vi "WILT Water Valve Control.vi"(0 "Valve Status":T7, 2 "Station Group":T4, 3 "Station Number":u32, 5 "Error In":errorcluster, 8 "Agilent Valve and Switch Locations":T3[](array[typedef])=[{"Channel"="301", "Station"="1", "Label"="Water Valve", "Agilent Station"="2", "Data"=0.0}, {"Channel"="302", "Station"="2", "Label"="Water Valve", "Agilent Station"="2", "Data"=0.0}, {"Channel"="303", "Station"="3", "Label"="Water Valve", "Agilent Station"="2", "Data"=0.0}, {"Channel"="304", "Station"="4", "Label"="Water Valve", "Agilent Station"="2", "Data"=0.0}, {"Channel"="305", "Station"="5", "Label"="Water Valve", "Agilent Station"="2", "Data"=0.0}, {"Channel"="306", "Station"="6", "Label"="Water Valve", "Agilent Station"="2", "Data"=0.0}, {"Channel"="307", "Station"="7", "Label"="Water Valve", "Agilent Station"="2", "Data"=0.0}, {"Channel"="308", "Station"="8", "Label"="Water Valve", "Agilent Station"="2", "Data"=0.0}, {"Channel"="309", "Station"="9", "Label"="Water Valve", "Agilent Station"="2", "Data"=0.0}, {"Channel"="310", "Station"="10", "Label"="Water Valve", "Agilent Station"="2", "Data"=0.0}, {"Channel"="311", "Station"="11", "Label"="Water Valve", "Agilent Station"="2", "Data"=0.0}, {"Channel"="312", "Station"="12", "Label"="Water Valve", "Agilent Station"="2", "Data"=0.0}, {"Channel"="313", "Station"="13", "Label"="Water Valve", "Agilent Station"="2", "Data"=0.0}, {"Channel"="314", "Station"="14", "Label"="Water Valve", "Agilent Station"="2", "Data"=0.0}, {"Channel"="315", "Station"="15", "Label"="Water Valve", "Agilent Station"="2", "Data"=0.0}, {"Channel"="316", "Station"="16", "Label"="Water Valve", "Agilent Station"="2", "Data"=0.0}, {"Channel"="317", "Station"="17", "Label"="Water Valve", "Agilent Station"="2", "Data"=0.0}, {"Channel"="318", "Station"="18", "Label"="Water Valve", "Agilent Station"="2", "Data"=0.0}, {"Channel"="319", "Station"="19", "Label"="Water Valve", "Agilent Station"="2", "Data"=0.0}, {"Channel"="320", "Station"="20", "Label"="Water Valve", "Agilent Station"="2", "Data"=0.0}, {"Channel"="101", "Station"="21", "Label"="Water Valve", "Agilent Station"="3", "Data"=0.0}, {"Channel"="102", "Station"="22", "Label"="Water Valve", "Agilent Station"="3", "Data"=0.0}, {"Channel"="103", "Station"="23", "Label"="Water Valve", "Agilent Station"="3", "Data"=0.0}, {"Channel"="104", "Station"="24", "Label"="Water Valve", "Agilent Station"="3", "Data"=0.0}, {"Channel"="105", "Station"="25", "Label"="Water Valve", "Agilent Station"="3", "Data"=0.0}, {"Channel"="106", "Station"="26", "Label"="Water Valve", "Agilent Station"="3", "Data"=0.0}, {"Channel"="107", "Station"="27", "Label"="Water Valve", "Agilent Station"="3", "Data"=0.0}, {"Channel"="108", "Station"="28", "Label"="Water Valve", "Agilent Station"="3", "Data"=0.0}, {"Channel"="109", "Station"="29", "Label"="Water Valve", "Agilent Station"="3", "Data"=0.0}, {"Channel"="110", "Station"="30", "Label"="Water Valve", "Agilent Station"="3", "Data"=0.0}, {"Channel"="111", "Station"="31", "Label"="Water Valve", "Agilent Station"="3", "Data"=0.0}, {"Channel"="112", "Station"="32", "Label"="Water Valve", "Agilent Station"="3", "Data"=0.0}, {"Channel"="101", "Station"="33", "Label"="Water Valve", "Agilent Station"="5", "Data"=0.0}, {"Channel"="102", "Station"="34", "Label"="Water Valve", "Agilent Station"="5", "Data"=0.0}, {"Channel"="103", "Station"="35", "Label"="Water Valve", "Agilent Station"="5", "Data"=0.0}, {"Channel"="104", "Station"="36", "Label"="Water Valve", "Agilent Station"="5", "Data"=0.0}, {"Channel"="105", "Station"="37", "Label"="Water Valve", "Agilent Station"="5", "Data"=0.0}, {"Channel"="106", "Station"="38", "Label"="Water Valve", "Agilent Station"="5", "Data"=0.0}, {"Channel"="107", "Station"="39", "Label"="Water Valve", "Agilent Station"="5", "Data"=0.0}, {"Channel"="108", "Station"="40", "Label"="Water Valve", "Agilent Station"="5", "Data"=0.0}, {"Channel"="109", "Station"="41", "Label"="Water Valve", "Agilent Station"="5", "Data"=0.0}, {"Channel"="110", "Station"="42", "Label"="Water Valve", "Agilent Station"="5", "Data"=0.0}, {"Channel"="111", "Station"="43", "Label"="Water Valve", "Agilent Station"="5", "Data"=0.0}, {"Channel"="112", "Station"="44", "Label"="Water Valve", "Agilent Station"="5", "Data"=0.0}, {"Channel"="113", "Station"="45", "Label"="Water Valve", "Agilent Station"="5", "Data"=0.0}, {"Channel"="114", "Station"="46", "Label"="Water Valve", "Agilent Station"="5", "Data"=0.0}, {"Channel"="115", "Station"="47", "Label"="Water Valve", "Agilent Station"="5", "Data"=0.0}, {"Channel"="116", "Station"="48", "Label"="Water Valve", "Agilent Station"="5", "Data"=0.0}, {"Channel"="117", "Station"="49", "Label"="Water Valve", "Agilent Station"="5", "Data"=0.0}, {"Channel"="118", "Station"="50", "Label"="Water Valve", "Agilent Station"="5", "Data"=0.0}, {"Channel"="119", "Station"="51", "Label"="Water Valve", "Agilent Station"="5", "Data"=0.0}, {"Channel"="120", "Station"="52", "Label"="Water Valve", "Agilent Station"="5", "Data"=0.0}, {"Channel"="201", "Station"="53", "Label"="Water Valve", "Agilent Station"="5", "Data"=0.0}, {"Channel"="202", "Station"="54", "Label"="Water Valve", "Agilent Station"="5", "Data"=0.0}, {"Channel"="203", "Station"="55", "Label"="Water Valve", "Agilent Station"="5", "Data"=0.0}, {"Channel"="204", "Station"="56", "Label"="Water Valve", "Agilent Station"="5", "Data"=0.0}, {"Channel"="301", "Station"="21", "Label"="Start Button", "Agilent Station"="5", "Data"=0.0}, {"Channel"="302", "Station"="22", "Label"="Start Button", "Agilent Station"="5", "Data"=0.0}, {"Channel"="303", "Station"="23", "Label"="Start Button", "Agilent Station"="5", "Data"=0.0}, {"Channel"="304", "Station"="24", "Label"="Start Button", "Agilent Station"="5", "Data"=0.0}, {"Channel"="305", "Station"="25", "Label"="Start Button", "Agilent Station"="5", "Data"=0.0}, {"Channel"="306", "Station"="26", "Label"="Start Button", "Agilent Station"="5", "Data"=0.0}, {"Channel"="307", "Station"="27", "Label"="Start Button", "Agilent Station"="5", "Data"=0.0}, {"Channel"="308", "Station"="28", "Label"="Start Button", "Agilent Station"="5", "Data"=0.0}, {"Channel"="309", "Station"="29", "Label"="Start Button", "Agilent Station"="5", "Data"=0.0}, {"Channel"="310", "Station"="30", "Label"="Start Button", "Agilent Station"="5", "Data"=0.0}, {"Channel"="311", "Station"="31", "Label"="Start Button", "Agilent Station"="5", "Data"=0.0}, {"Channel"="312", "Station"="32", "Label"="Start Button", "Agilent Station"="5", "Data"=0.0}, {"Channel"="101", "Station"="33", "Label"="Start Button", "Agilent Station"="7", "Data"=0.0}, {"Channel"="102", "Station"="34", "Label"="Start Button", "Agilent Station"="7", "Data"=0.0}, {"Channel"="103", "Station"="35", "Label"="Start Button", "Agilent Station"="7", "Data"=0.0}, {"Channel"="104", "Station"="36", "Label"="Start Button", "Agilent Station"="7", "Data"=0.0}, {"Channel"="105", "Station"="37", "Label"="Start Button", "Agilent Station"="7", "Data"=0.0}, {"Channel"="106", "Station"="38", "Label"="Start Button", "Agilent Station"="7", "Data"=0.0}, {"Channel"="107", "Station"="39", "Label"="Start Button", "Agilent Station"="7", "Data"=0.0}, {"Channel"="108", "Station"="40", "Label"="Start Button", "Agilent Station"="7", "Data"=0.0}, {"Channel"="109", "Station"="41", "Label"="Start Button", "Agilent Station"="7", "Data"=0.0}, {"Channel"="110", "Station"="42", "Label"="Start Button", "Agilent Station"="7", "Data"=0.0}, {"Channel"="111", "Station"="43", "Label"="Start Button", "Agilent Station"="7", "Data"=0.0}, {"Channel"="112", "Station"="44", "Label"="Start Button", "Agilent Station"="7", "Data"=0.0}, {"Channel"="113", "Station"="45", "Label"="Start Button", "Agilent Station"="7", "Data"=0.0}, {"Channel"="114", "Station"="46", "Label"="Start Button", "Agilent Station"="7", "Data"=0.0}, {"Channel"="115", "Station"="47", "Label"="Start Button", "Agilent Station"="7", "Data"=0.0}, {"Channel"="116", "Station"="48", "Label"="Start Button", "Agilent Station"="7", "Data"=0.0}, {"Channel"="117", "Station"="49", "Label"="Start Button", "Agilent Station"="7", "Data"=0.0}, {"Channel"="118", "Station"="50", "Label"="Start Button", "Agilent Station"="7", "Data"=0.0}, {"Channel"="119", "Station"="51", "Label"="Start Button", "Agilent Station"="7", "Data"=0.0}, {"Channel"="120", "Station"="52", "Label"="Start Button", "Agilent Station"="7", "Data"=0.0}, {"Channel"="201", "Station"="53", "Label"="Start Button", "Agilent Station"="7", "Data"=0.0}, {"Channel"="202", "Station"="54", "Label"="Start Button", "Agilent Station"="7", "Data"=0.0}, {"Channel"="203", "Station"="55", "Label"="Start Button", "Agilent Station"="7", "Data"=0.0}, {"Channel"="204", "Station"="56", "Label"="Start Button", "Agilent Station"="7", "Data"=0.0}], 9 "Step 3 Input in":T5, 11 "Day/Night Cycle":T2, 13 "Semaphore":T1[](array[typedef])) -> (14 "Step 3 Input out":T5, 19 "Error Out":errorcluster)   [LabVIEW 2016]
uses:
  Type Definitions/WILT Water Valve Control.ctl
  Type Definitions/WILT Station Test State Cluster.ctl
  Type Definitions/WILT Dryer Test State.ctl
  Type Definitions/WILT Room Location.ctl
  Type Definitions/WILT Agilent Channel Definition.ctl
  Type Definitions/WILT Day Night Cycle Enum.ctl
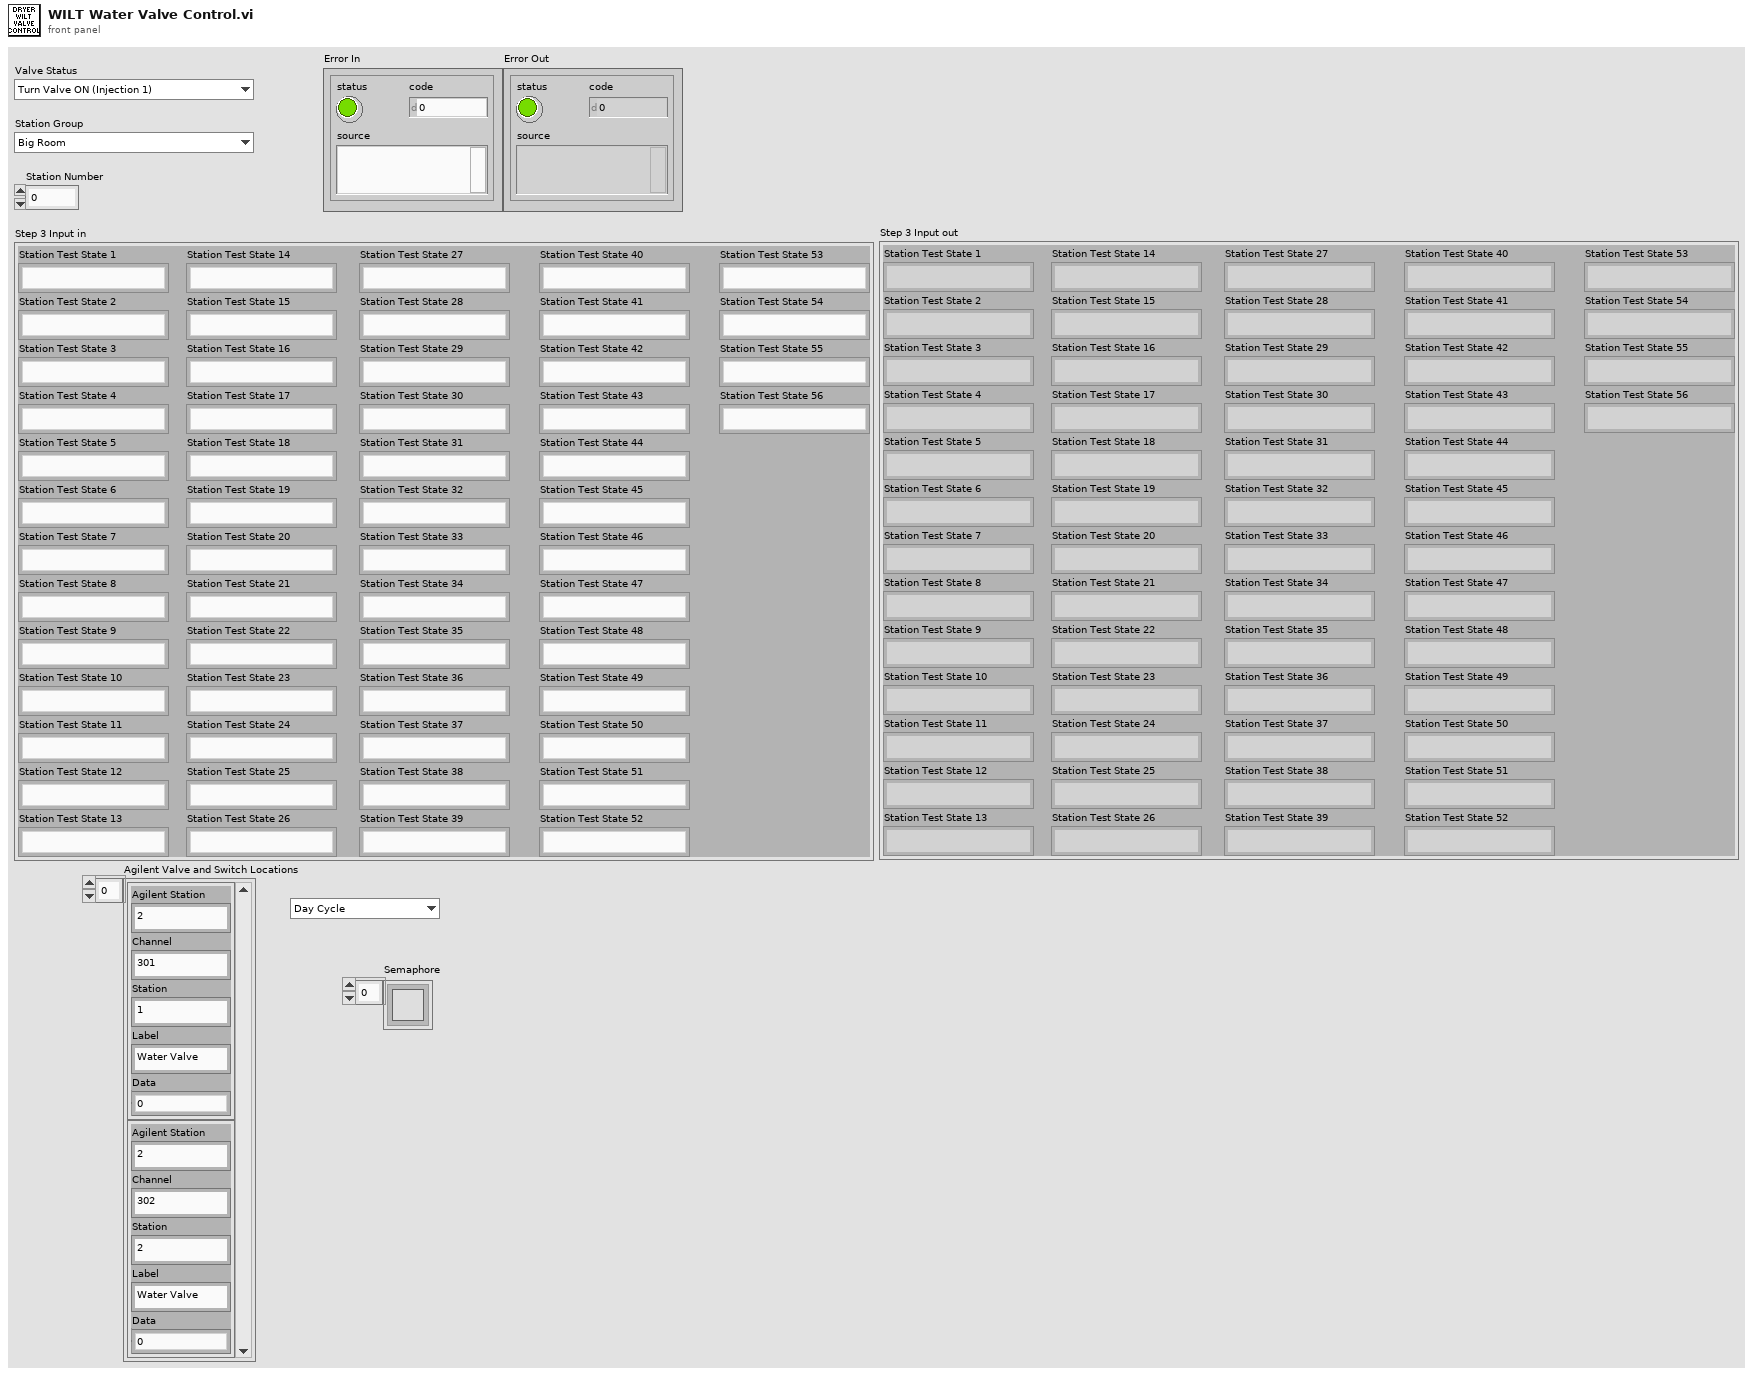
[diagram p1: front panel]
types:
  T1 = typedef "Semaphore RefNum" = refnum<k1>
  T2 = typedef "WILT Day Night Cycle Enum.ctl" = enum16{"Day Cycle", "Night Cycle", "Day Cycle (No Water)"}
  T3 = typedef "WILT Agilent Channel Definition.ctl" = cluster{"Channel":string, "Station":string, "Label":string, "Agilent Station":string, "Data":dbl}
  T4 = typedef "WILT Room Location.ctl" = enum16{"Big Room", "Remote Stations"}
  T5 = typedef "WILT Station Test State Cluster.ctl" = cluster{"Station Test State 1":T6, "Station Test State 2":T6, "Station Test State 3":T6, "Station Test State 4":T6, "Station Test State 5":T6, "Station Test State 6":T6, "Station Test State 7":T6, "Station Test State 8":T6, "Station Test State 9":T6, "Station Test State 10":T6, "Station Test State 11":T6, "Station Test State 12":T6, "Station Test State 13":T6, "Station Test State 14":T6, "Station Test State 15":T6, "Station Test State 16":T6, "Station Test State 17":T6, "Station Test State 18":T6, "Station Test State 19":T6, "Station Test State 20":T6, "Station Test State 21":T6, "Station Test State 22":T6, "Station Test State 23":T6, "Station Test State 24":T6, "Station Test State 25":T6, "Station Test State 26":T6, "Station Test State 27":T6, "Station Test State 28":T6, "Station Test State 29":T6, "Station Test State 30":T6, "Station Test State 31":T6, "Station Test State 32":T6, "Station Test State 33":T6, "Station Test State 34":T6, "Station Test State 35":T6, "Station Test State 36":T6, "Station Test State 37":T6, "Station Test State 38":T6, "Station Test State 39":T6, "Station Test State 40":T6, "Station Test State 41":T6, "Station Test State 42":T6, "Station Test State 43":T6, "Station Test State 44":T6, "Station Test State 45":T6, "Station Test State 46":T6, "Station Test State 47":T6, "Station Test State 48":T6, "Station Test State 49":T6, "Station Test State 50":T6, "Station Test State 51":T6, "Station Test State 52":T6, "Station Test State 53":T6, "Station Test State 54":T6, "Station Test State 55":T6, "Station Test State 56":T6}
  T6 = typedef "WILT Dryer Test State.ctl" = enum16{"No Serial Number", "Waiting for Dryer To Start", "Drying Clothes", "Water Injection 1 (On)", "Water Injection 1 Timer", "Water Injection 1 (Off)", "Pause Dryer", "Sending Start Stop CMD", "Pause Dryer 2", "Sending Start Stop CMD 2", "Drying Clothes 2", "Water Injection 2 (On)", "Water Injection 2 Timer", "Water Injection 2 (Off)", "Drying Clothes 3", "Cooling Down", "Sending Start Stop CMD 3", "Increment Cycle"}
  T7 = typedef "WILT Water Valve Control.ctl" = enum16{"Turn Valve ON (Injection 1)", "Turn Valve OFF (Injection 1)", "Turn Valve ON (Injection 2)", "Turn Valve OFF (Injection 2)"}
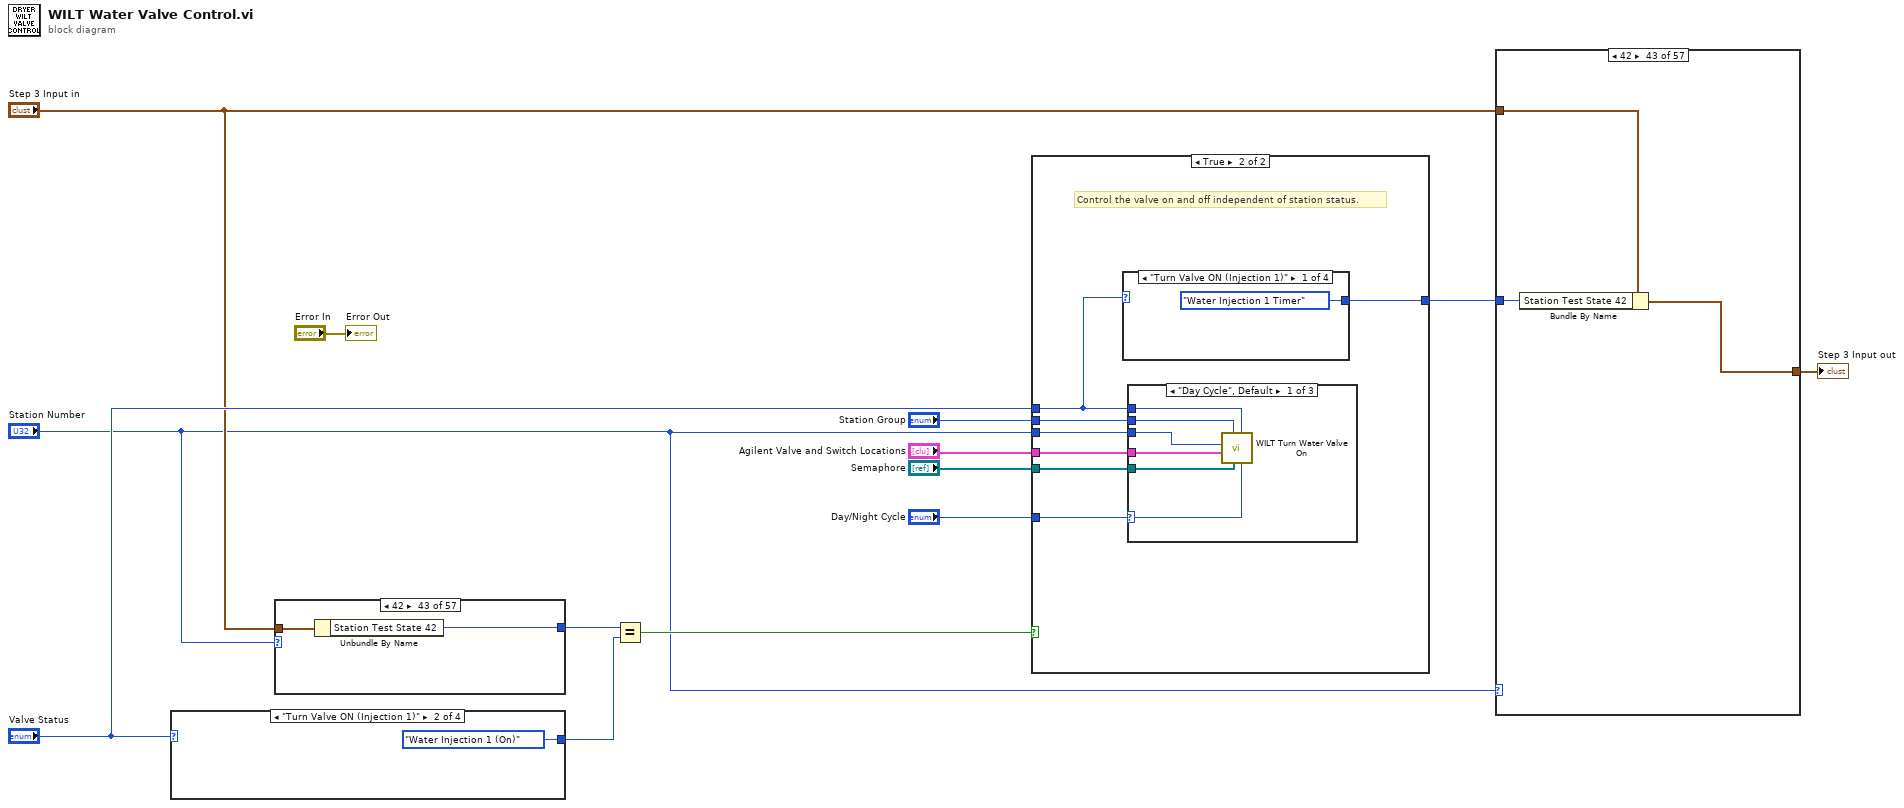
[diagram p0: block diagram]
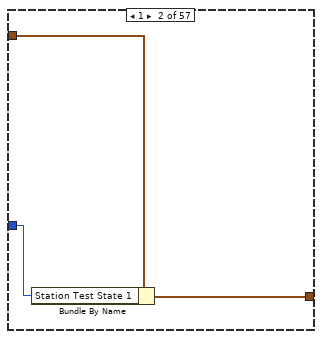
[diagram p3: hidden frame]
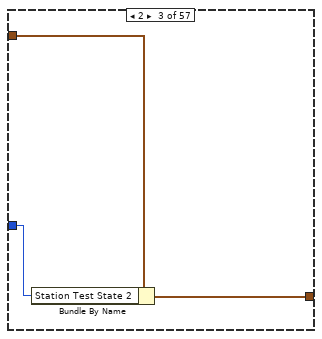
[diagram p4: hidden frame]
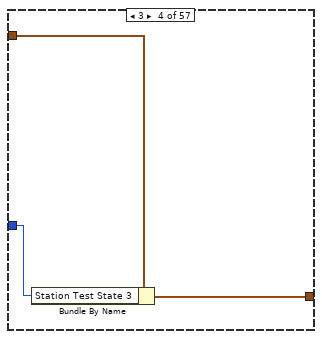
[diagram p5: hidden frame]
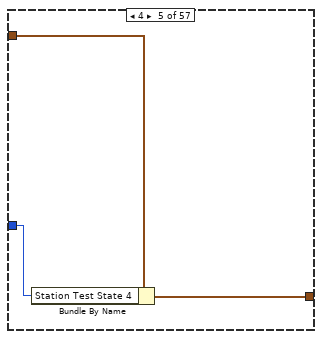
[diagram p6: hidden frame]
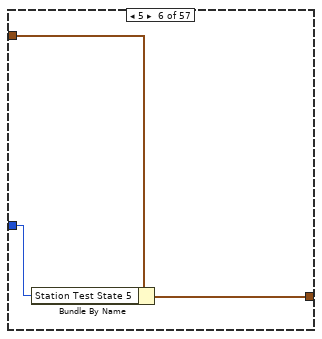
[diagram p7: hidden frame]
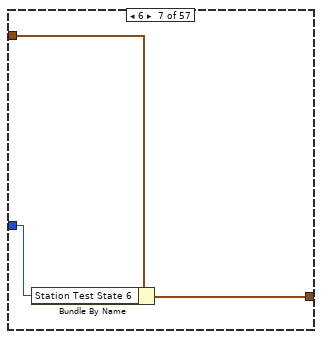
[diagram p8: hidden frame]
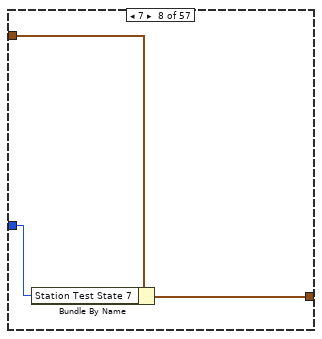
[diagram p9: hidden frame]
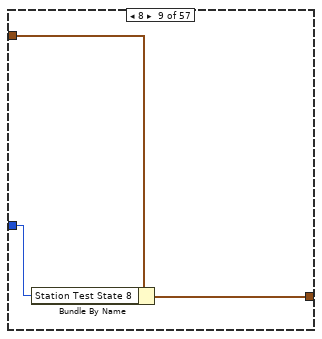
[diagram p10: hidden frame]
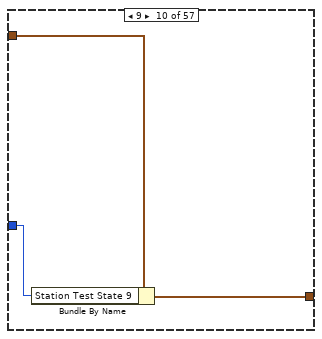
[diagram p11: hidden frame]
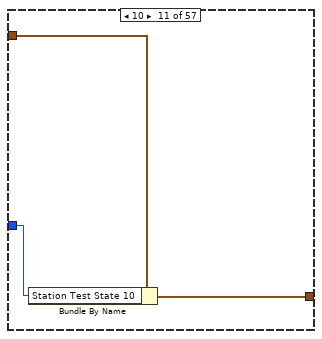
[diagram p12: hidden frame]
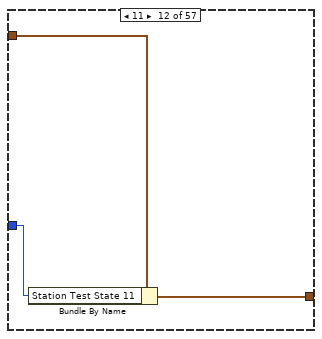
[diagram p13: hidden frame]
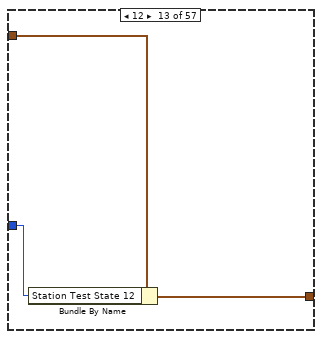
[diagram p14: hidden frame]
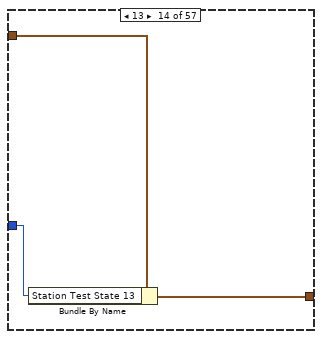
[diagram p15: hidden frame]
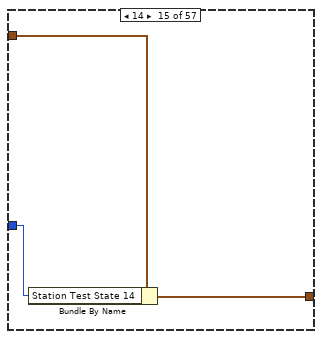
[diagram p16: hidden frame]
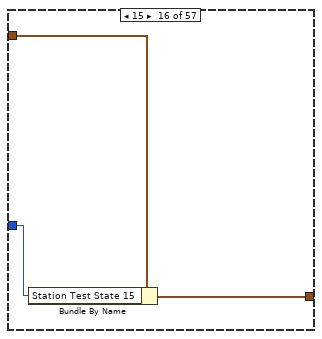
[diagram p17: hidden frame]
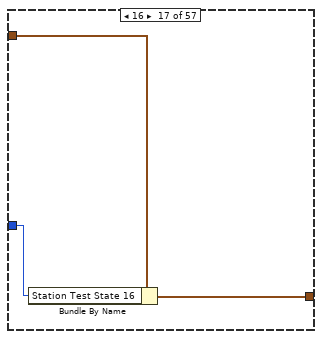
[diagram p18: hidden frame]
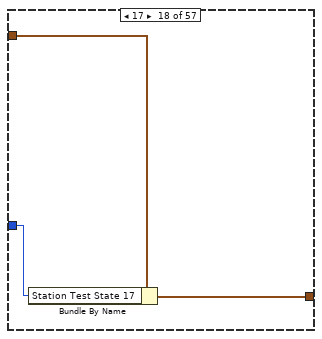
[diagram p19: hidden frame]
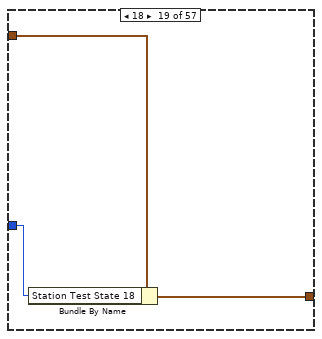
[diagram p20: hidden frame]
diagram:
  n1 = case shown="\"Turn Valve ON (Injection 1)\"" "Valve Status" {
    tunnel: [WILT_Dryer_Test_State."Water Injection 1 (Off)" ("y") WILT_Dryer_Test_State."Water Injection 1 (On)" ("y") WILT_Dryer_Test_State."Water Injection 2 (On)" ("y") WILT_Dryer_Test_State."Water Injection 2 (Off)" ("y")] -> w10
    frame "Turn Valve OFF (Injection 1)", Default {
    }
    frame "Turn Valve ON (Injection 1)" {
    }
    frame "Turn Valve ON (Injection 2)" {
    }
    frame "Turn Valve OFF (Injection 2)" {
    }
  }
  n2 = case shown="42" "Station Number" {
    tunnel: "Step 3 Input in" -> [_ w20 w22 w24 w26 w28 w30 w32 w34 w36 w38 w40 w42 w44 w46 w48 w50 w52 w54 w56 w58 w60 w62 w64 w66 w68 w70 w72 w74 w76 w78 w80 w82 w84 w86 w88 w90 w92 w94 w96 w98 w100 w102 w104 w106 w108 w110 w112 w114 w116 w118 w120 w122 w124 w126 w128 w130]
    tunnel: [WILT_Dryer_Test_State."No Serial Number" ("Station Test State 56") w19 w21 w23 w25 w27 w29 w31 w33 w35 w37 w39 w41 w43 w45 w47 w49 w51 w53 w55 w57 w59 w61 w63 w65 w67 w69 w71 w73 w75 w77 w79 w81 w83 w85 w87 w89 w91 w93 w95 w97 w99 w101 w103 w105 w107 w109 w111 w113 w115 w117 w119 w121 w123 w125 w127 w129] -> w9
    frame 0, Default {
      # "This is not a station.\nDo nothing"
    }
    frame 1 {
      n3 = Unbundle By Name(w20) -> ("Station Test State 1"=w19:T6)
    }
    frame 2 {
      n4 = Unbundle By Name(w22) -> ("Station Test State 2"=w21:T6)
    }
    frame 3 {
      n5 = Unbundle By Name(w24) -> ("Station Test State 3"=w23:T6)
    }
    frame 4 {
      n6 = Unbundle By Name(w26) -> ("Station Test State 4"=w25:T6)
    }
    frame 5 {
      n7 = Unbundle By Name(w28) -> ("Station Test State 5"=w27:T6)
    }
    frame 6 {
      n8 = Unbundle By Name(w30) -> ("Station Test State 6"=w29:T6)
    }
    frame 7 {
      n9 = Unbundle By Name(w32) -> ("Station Test State 7"=w31:T6)
    }
    frame 8 {
      n10 = Unbundle By Name(w34) -> ("Station Test State 8"=w33:T6)
    }
    frame 9 {
      n11 = Unbundle By Name(w36) -> ("Station Test State 9"=w35:T6)
    }
    frame 10 {
      n12 = Unbundle By Name(w38) -> ("Station Test State 10"=w37:T6)
    }
    frame 11 {
      n13 = Unbundle By Name(w40) -> ("Station Test State 11"=w39:T6)
    }
    frame 12 {
      n14 = Unbundle By Name(w42) -> ("Station Test State 12"=w41:T6)
    }
    frame 13 {
      n15 = Unbundle By Name(w44) -> ("Station Test State 13"=w43:T6)
    }
    frame 14 {
      n16 = Unbundle By Name(w46) -> ("Station Test State 14"=w45:T6)
    }
    frame 15 {
      n17 = Unbundle By Name(w48) -> ("Station Test State 15"=w47:T6)
    }
    frame 16 {
      n18 = Unbundle By Name(w50) -> ("Station Test State 16"=w49:T6)
    }
    frame 17 {
      n19 = Unbundle By Name(w52) -> ("Station Test State 17"=w51:T6)
    }
    frame 18 {
      n20 = Unbundle By Name(w54) -> ("Station Test State 18"=w53:T6)
    }
    frame 19 {
      n21 = Unbundle By Name(w56) -> ("Station Test State 19"=w55:T6)
    }
    frame 20 {
      n22 = Unbundle By Name(w58) -> ("Station Test State 20"=w57:T6)
    }
    frame 21 {
      n23 = Unbundle By Name(w60) -> ("Station Test State 21"=w59:T6)
    }
    frame 22 {
      n24 = Unbundle By Name(w62) -> ("Station Test State 22"=w61:T6)
    }
    frame 23 {
      n25 = Unbundle By Name(w64) -> ("Station Test State 23"=w63:T6)
    }
    frame 24 {
      n26 = Unbundle By Name(w66) -> ("Station Test State 24"=w65:T6)
    }
    frame 25 {
      n27 = Unbundle By Name(w68) -> ("Station Test State 25"=w67:T6)
    }
    frame 26 {
      n28 = Unbundle By Name(w70) -> ("Station Test State 26"=w69:T6)
    }
    frame 27 {
      n29 = Unbundle By Name(w72) -> ("Station Test State 27"=w71:T6)
    }
    frame 28 {
      n30 = Unbundle By Name(w74) -> ("Station Test State 28"=w73:T6)
    }
    frame 29 {
      n31 = Unbundle By Name(w76) -> ("Station Test State 29"=w75:T6)
    }
    frame 30 {
      n32 = Unbundle By Name(w78) -> ("Station Test State 30"=w77:T6)
    }
    frame 31 {
      n33 = Unbundle By Name(w80) -> ("Station Test State 31"=w79:T6)
    }
    frame 32 {
      n34 = Unbundle By Name(w82) -> ("Station Test State 32"=w81:T6)
    }
    frame 33 {
      n35 = Unbundle By Name(w84) -> ("Station Test State 33"=w83:T6)
    }
    frame 34 {
      n36 = Unbundle By Name(w86) -> ("Station Test State 34"=w85:T6)
    }
    frame 35 {
      n37 = Unbundle By Name(w88) -> ("Station Test State 35"=w87:T6)
    }
    frame 36 {
      n38 = Unbundle By Name(w90) -> ("Station Test State 36"=w89:T6)
    }
    frame 37 {
      n39 = Unbundle By Name(w92) -> ("Station Test State 37"=w91:T6)
    }
    frame 38 {
      n40 = Unbundle By Name(w94) -> ("Station Test State 38"=w93:T6)
    }
    frame 39 {
      n41 = Unbundle By Name(w96) -> ("Station Test State 39"=w95:T6)
    }
    frame 40 {
      n42 = Unbundle By Name(w98) -> ("Station Test State 40"=w97:T6)
    }
    frame 41 {
      n43 = Unbundle By Name(w100) -> ("Station Test State 41"=w99:T6)
    }
    frame 42 {
      n44 = Unbundle By Name(w102) -> ("Station Test State 42"=w101:T6)
    }
    frame 43 {
      n45 = Unbundle By Name(w104) -> ("Station Test State 43"=w103:T6)
    }
    frame 44 {
      n46 = Unbundle By Name(w106) -> ("Station Test State 44"=w105:T6)
    }
    frame 45 {
      n47 = Unbundle By Name(w108) -> ("Station Test State 45"=w107:T6)
    }
    frame 46 {
      n48 = Unbundle By Name(w110) -> ("Station Test State 46"=w109:T6)
    }
    frame 47 {
      n49 = Unbundle By Name(w112) -> ("Station Test State 47"=w111:T6)
    }
    frame 48 {
      n50 = Unbundle By Name(w114) -> ("Station Test State 48"=w113:T6)
    }
    frame 49 {
      n51 = Unbundle By Name(w116) -> ("Station Test State 49"=w115:T6)
    }
    frame 50 {
      n52 = Unbundle By Name(w118) -> ("Station Test State 50"=w117:T6)
    }
    frame 51 {
      n53 = Unbundle By Name(w120) -> ("Station Test State 51"=w119:T6)
    }
    frame 52 {
      n54 = Unbundle By Name(w122) -> ("Station Test State 52"=w121:T6)
    }
    frame 53 {
      n55 = Unbundle By Name(w124) -> ("Station Test State 53"=w123:T6)
    }
    frame 54 {
      n56 = Unbundle By Name(w126) -> ("Station Test State 54"=w125:T6)
    }
    frame 55 {
      n57 = Unbundle By Name(w128) -> ("Station Test State 55"=w127:T6)
    }
    frame 56 {
      n58 = Unbundle By Name(w130) -> ("Station Test State 56"=w129:T6)
    }
  }
  n59 = Equal?(x=w9, y=w10) -> (x = y?=w11:bool)
  n60 = case shown="True" w11 {
    tunnel: "Station Number" -> [_ w138]
    tunnel: "Valve Status" -> [_ w135]
    tunnel: "Station Group" -> [_ w137]
    tunnel: [WILT_Dryer_Test_State."Waiting for Dryer To Start" ("Station Test State 56") w136] -> w7
    tunnel: "Agilent Valve and Switch Locations" -> [_ w134]
    tunnel: "Day/Night Cycle" -> [_ w133]
    tunnel: "Semaphore" -> [_ w132]
    frame False {
    }
    frame True {
      # "Control the valve on and off independent of station status."
      n61 = case shown="\"Turn Valve ON (Injection 1)\"" w135 {
        tunnel: [WILT_Dryer_Test_State."Water Injection 1 Timer" ("Station Test State 56") WILT_Dryer_Test_State."Pause Dryer" ("Station Test State 56") WILT_Dryer_Test_State."Water Injection 2 Timer" ("Station Test State 56") WILT_Dryer_Test_State."Drying Clothes 3" ("Station Test State 56")] -> w136
        frame "Turn Valve ON (Injection 1)" {
        }
        frame "Turn Valve OFF (Injection 1)", Default {
        }
        frame "Turn Valve ON (Injection 2)" {
        }
        frame "Turn Valve OFF (Injection 2)" {
        }
      }
      n62 = case shown="\"Day Cycle\", Default" w133 {
        selector: w133 -> [w139 _ w149]
        tunnel: w138 -> [w144 _ w147]
        tunnel: w137 -> [w143 _ w146]
        tunnel: w135 -> [w142 _ w145]
        tunnel: w134 -> [w141 _ w148]
        tunnel: w132 -> [w140 _ w150]
        frame "Day Cycle", Default {
          n63 = call "WILT Turn Water Valve On.vi"("Day/Night Cycle"=w139, "Valve Status"=w142, "Semaphore"=w140, "Station Group"=w143, "Agilent Valve and Switch Locations"=w141, "Station Index"=w144) -> ()  [unwired: 5 in, 1 out]
        }
        frame "Night Cycle" {
        }
        frame "Day Cycle (No Water)" {
          n64 = call "WILT Turn Water Valve On.vi"("Day/Night Cycle"=w149, "Valve Status"=w145, "Semaphore"=w150, "Station Group"=w146, "Agilent Valve and Switch Locations"=w148, "Station Index"=w147) -> ()  [unwired: 5 in, 1 out]
        }
      }
    }
  }
  n65 = case shown="42" "Station Number" {
    tunnel: "Step 3 Input in" -> [w155 w158 w161 w164 w167 w170 w173 w176 w179 w182 w185 w188 w191 w194 w197 w200 w203 w206 w209 w212 w215 w218 w221 w224 w227 w230 w233 w236 w239 w242 w245 w248 w251 w254 w257 w260 w263 w266 w269 w272 w275 w278 w281 w284 w287 w290 w293 w296 w299 w302 w305 w308 w311 w314 w317 w320 w323]
    tunnel: w7 -> [_ w157 w159 w162 w165 w168 w171 w174 w177 w180 w183 w186 w189 w192 w195 w198 w201 w204 w207 w210 w213 w216 w219 w222 w225 w228 w231 w234 w237 w240 w243 w246 w249 w252 w255 w258 w261 w264 w267 w270 w273 w276 w279 w282 w285 w288 w291 w294 w297 w300 w303 w306 w309 w312 w315 w318 w321]
    tunnel: [w155 w156 w160 w163 w166 w169 w172 w175 w178 w181 w184 w187 w190 w193 w196 w199 w202 w205 w208 w211 w214 w217 w220 w223 w226 w229 w232 w235 w238 w241 w244 w247 w250 w253 w256 w259 w262 w265 w268 w271 w274 w277 w280 w283 w286 w289 w292 w295 w298 w301 w304 w307 w310 w313 w316 w319 w322] -> w5
    frame 0, Default {
      # "Not a valid station. Do nothing"
    }
    frame 1 {
      n66 = Bundle By Name(cluster=w158, "Station Test State 1"=w157) -> (w156:T5)
    }
    frame 2 {
      n67 = Bundle By Name(cluster=w161, "Station Test State 2"=w159) -> (w160:T5)
    }
    frame 3 {
      n68 = Bundle By Name(cluster=w164, "Station Test State 3"=w162) -> (w163:T5)
    }
    frame 4 {
      n69 = Bundle By Name(cluster=w167, "Station Test State 4"=w165) -> (w166:T5)
    }
    frame 5 {
      n70 = Bundle By Name(cluster=w170, "Station Test State 5"=w168) -> (w169:T5)
    }
    frame 6 {
      n71 = Bundle By Name(cluster=w173, "Station Test State 6"=w171) -> (w172:T5)
    }
    frame 7 {
      n72 = Bundle By Name(cluster=w176, "Station Test State 7"=w174) -> (w175:T5)
    }
    frame 8 {
      n73 = Bundle By Name(cluster=w179, "Station Test State 8"=w177) -> (w178:T5)
    }
    frame 9 {
      n74 = Bundle By Name(cluster=w182, "Station Test State 9"=w180) -> (w181:T5)
    }
    frame 10 {
      n75 = Bundle By Name(cluster=w185, "Station Test State 10"=w183) -> (w184:T5)
    }
    frame 11 {
      n76 = Bundle By Name(cluster=w188, "Station Test State 11"=w186) -> (w187:T5)
    }
    frame 12 {
      n77 = Bundle By Name(cluster=w191, "Station Test State 12"=w189) -> (w190:T5)
    }
    frame 13 {
      n78 = Bundle By Name(cluster=w194, "Station Test State 13"=w192) -> (w193:T5)
    }
    frame 14 {
      n79 = Bundle By Name(cluster=w197, "Station Test State 14"=w195) -> (w196:T5)
    }
    frame 15 {
      n80 = Bundle By Name(cluster=w200, "Station Test State 15"=w198) -> (w199:T5)
    }
    frame 16 {
      n81 = Bundle By Name(cluster=w203, "Station Test State 16"=w201) -> (w202:T5)
    }
    frame 17 {
      n82 = Bundle By Name(cluster=w206, "Station Test State 17"=w204) -> (w205:T5)
    }
    frame 18 {
      n83 = Bundle By Name(cluster=w209, "Station Test State 18"=w207) -> (w208:T5)
    }
    frame 19 {
      n84 = Bundle By Name(cluster=w212, "Station Test State 19"=w210) -> (w211:T5)
    }
    frame 20 {
      n85 = Bundle By Name(cluster=w215, "Station Test State 20"=w213) -> (w214:T5)
    }
    frame 21 {
      n86 = Bundle By Name(cluster=w218, "Station Test State 21"=w216) -> (w217:T5)
    }
    frame 22 {
      n87 = Bundle By Name(cluster=w221, "Station Test State 22"=w219) -> (w220:T5)
    }
    frame 23 {
      n88 = Bundle By Name(cluster=w224, "Station Test State 23"=w222) -> (w223:T5)
    }
    frame 24 {
      n89 = Bundle By Name(cluster=w227, "Station Test State 24"=w225) -> (w226:T5)
    }
    frame 25 {
      n90 = Bundle By Name(cluster=w230, "Station Test State 25"=w228) -> (w229:T5)
    }
    frame 26 {
      n91 = Bundle By Name(cluster=w233, "Station Test State 26"=w231) -> (w232:T5)
    }
    frame 27 {
      n92 = Bundle By Name(cluster=w236, "Station Test State 27"=w234) -> (w235:T5)
    }
    frame 28 {
      n93 = Bundle By Name(cluster=w239, "Station Test State 28"=w237) -> (w238:T5)
    }
    frame 29 {
      n94 = Bundle By Name(cluster=w242, "Station Test State 29"=w240) -> (w241:T5)
    }
    frame 30 {
      n95 = Bundle By Name(cluster=w245, "Station Test State 30"=w243) -> (w244:T5)
    }
    frame 31 {
      n96 = Bundle By Name(cluster=w248, "Station Test State 31"=w246) -> (w247:T5)
    }
    frame 32 {
      n97 = Bundle By Name(cluster=w251, "Station Test State 32"=w249) -> (w250:T5)
    }
    frame 33 {
      n98 = Bundle By Name(cluster=w254, "Station Test State 33"=w252) -> (w253:T5)
    }
    frame 34 {
      n99 = Bundle By Name(cluster=w257, "Station Test State 34"=w255) -> (w256:T5)
    }
    frame 35 {
      n100 = Bundle By Name(cluster=w260, "Station Test State 35"=w258) -> (w259:T5)
    }
    frame 36 {
      n101 = Bundle By Name(cluster=w263, "Station Test State 36"=w261) -> (w262:T5)
    }
    frame 37 {
      n102 = Bundle By Name(cluster=w266, "Station Test State 37"=w264) -> (w265:T5)
    }
    frame 38 {
      n103 = Bundle By Name(cluster=w269, "Station Test State 38"=w267) -> (w268:T5)
    }
    frame 39 {
      n104 = Bundle By Name(cluster=w272, "Station Test State 39"=w270) -> (w271:T5)
    }
    frame 40 {
      n105 = Bundle By Name(cluster=w275, "Station Test State 40"=w273) -> (w274:T5)
    }
    frame 41 {
      n106 = Bundle By Name(cluster=w278, "Station Test State 41"=w276) -> (w277:T5)
    }
    frame 42 {
      n107 = Bundle By Name(cluster=w281, "Station Test State 42"=w279) -> (w280:T5)
    }
    frame 43 {
      n108 = Bundle By Name(cluster=w284, "Station Test State 43"=w282) -> (w283:T5)
    }
    frame 44 {
      n109 = Bundle By Name(cluster=w287, "Station Test State 44"=w285) -> (w286:T5)
    }
    frame 45 {
      n110 = Bundle By Name(cluster=w290, "Station Test State 45"=w288) -> (w289:T5)
    }
    frame 46 {
      n111 = Bundle By Name(cluster=w293, "Station Test State 46"=w291) -> (w292:T5)
    }
    frame 47 {
      n112 = Bundle By Name(cluster=w296, "Station Test State 47"=w294) -> (w295:T5)
    }
    frame 48 {
      n113 = Bundle By Name(cluster=w299, "Station Test State 48"=w297) -> (w298:T5)
    }
    frame 49 {
      n114 = Bundle By Name(cluster=w302, "Station Test State 49"=w300) -> (w301:T5)
    }
    frame 50 {
      n115 = Bundle By Name(cluster=w305, "Station Test State 50"=w303) -> (w304:T5)
    }
    frame 51 {
      n116 = Bundle By Name(cluster=w308, "Station Test State 51"=w306) -> (w307:T5)
    }
    frame 52 {
      n117 = Bundle By Name(cluster=w311, "Station Test State 52"=w309) -> (w310:T5)
    }
    frame 53 {
      n118 = Bundle By Name(cluster=w314, "Station Test State 53"=w312) -> (w313:T5)
    }
    frame 54 {
      n119 = Bundle By Name(cluster=w317, "Station Test State 54"=w315) -> (w316:T5)
    }
    frame 55 {
      n120 = Bundle By Name(cluster=w320, "Station Test State 55"=w318) -> (w319:T5)
    }
    frame 56 {
      n121 = Bundle By Name(cluster=w323, "Station Test State 56"=w321) -> (w322:T5)
    }
  }
  "Step 3 Input out" <- w5
  "Error Out" <- "Error In"
